vi "save_wl_to_config.vi"(6 "wavelength \n(calibration value)":dbl[](array[numeric]), 9 "best fit parameters":dbl[](array[numeric]), 10 "appended path":path, 11 "pix":u16[](array[numeric])) -> (0 "error out":errorcluster)   [LabVIEW 2019]
uses:
  <vilib>/Utility/config.llb/Write Key (Double).vi
  <vilib>/Utility/config.llb/Write Key (String).vi
  <vilib>/Utility/config.llb/NI_LVConfig.lvlib
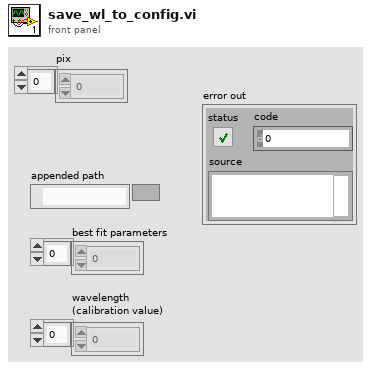
[diagram p1: front panel]
types:
  T1 = typedef "NI_LVConfig.lvlib/Config Data RefNum.ctl" = refnum<k1>
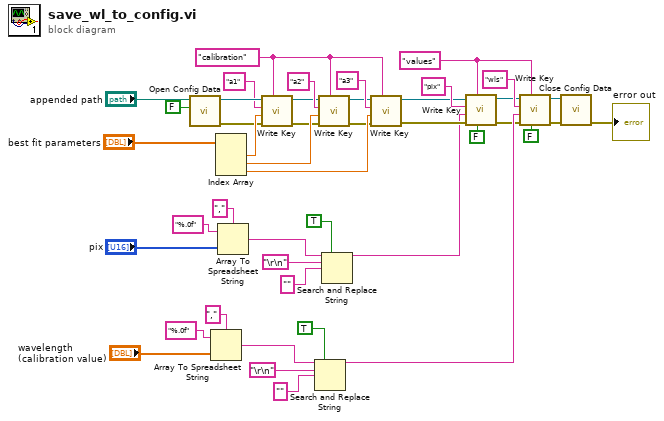
[diagram p0: block diagram]
diagram:
  w28 = "values" ("section")
  w14 = "calibration" ("section")
  n1 = call <vilib>:"Open Config Data.vi"("create file if necessary (T)"=FALSE, "configuration file path"="appended path") -> ("error out"=w12:errorcluster, "refnum"=w11:T1)  [unwired: 7 in, 1 out]
  n2 = Array To Spreadsheet String(delimiter (Tab)=",", array="wavelength \n(calibration value)", 3:"%.0f" ("format string")) -> (spreadsheet string=w40:string)
  n3 = Index Array(array="best fit parameters") -> (element #1=w13:dbl, element #2=w21:dbl, element #3=w22:dbl)  [unwired: 3 in]
  n4 = Array To Spreadsheet String(delimiter (Tab)=",", array="pix", 3:"%.0f" ("format string")) -> (spreadsheet string=w3:string)
  n5 = call-poly <vilib>:"Write Key.vi"("section"=w14, "error in (no error)"=w12, "value"=w13, "key"="a1", "refnum"=w11) -> ("error out"=w18:errorcluster, "refnum out"=w15:T1)  [unwired: 4 in, 1 out]
  n6 = Search and Replace String(replace all?=TRUE ("replace all? (F)"), input string=w40, search string="\r\n", replace string="" ("replace string (\"\")")) -> (result string=w42:string)  [unwired: 4 in, 3 out]
  n7 = call-poly <vilib>:"Write Key.vi"("section"=w14, "error in (no error)"=w18, "value"=w21, "key"="a2", "refnum"=w15) -> ("error out"=w17:errorcluster, "refnum out"=w16:T1)  [unwired: 4 in, 1 out]
  n8 = Search and Replace String(replace all?=TRUE ("replace all? (F)"), input string=w3, search string="\r\n", replace string="" ("replace string (\"\")")) -> (result string=w4:string)  [unwired: 4 in, 3 out]
  n9 = call-poly <vilib>:"Write Key.vi"("section"=w14, "error in (no error)"=w17, "value"=w22, "key"="a3", "refnum"=w16) -> ("error out"=w24:errorcluster, "refnum out"=w23:T1)  [unwired: 4 in, 1 out]
  n10 = call-poly <vilib>:"Write Key.vi"("write raw string? (F)"=FALSE, "section"=w28, "error in (no error)"=w24, "value"=w4, "key"="pix", "refnum"=w23) -> ("error out"=w27:errorcluster, "refnum out"=w26:T1)  [unwired: 3 in, 1 out]
  n11 = call-poly <vilib>:"Write Key.vi"("write raw string? (F)"=FALSE, "section"=w28, "error in (no error)"=w27, "value"=w42, "key"="wls", "refnum"=w26) -> ("error out"=w35:errorcluster, "refnum out"=w38:T1)  [unwired: 3 in, 1 out]
  n12 = call <vilib>:"Close Config Data.vi"("error in (no error)"=w35, "refnum"=w38) -> ("error out"=→"error out":errorcluster)  [unwired: 8 in, 1 out]
